vi "Smoothen Noise below Threshold.vi"(8 "Error In":errorcluster, 9 "Smoothing Width":dbl=1.0, 10 "Noise Threshold":dbl, 11 "Function in":dbl[](array[numeric])) -> (0 "Error Out":errorcluster, 3 "Function out":dbl[](array[numeric]))   [LabVIEW 2021, in "Arrays.lvlib"]
uses:
  Arrays.lvlib
  Linear Ramp End Options.ctl
  e7203b3f-f00a-46c5-81ee-9b5c31ab6268.vi
panel:
  out "Support Size":i32
  out "Waveform Graph":dbl[](graph)
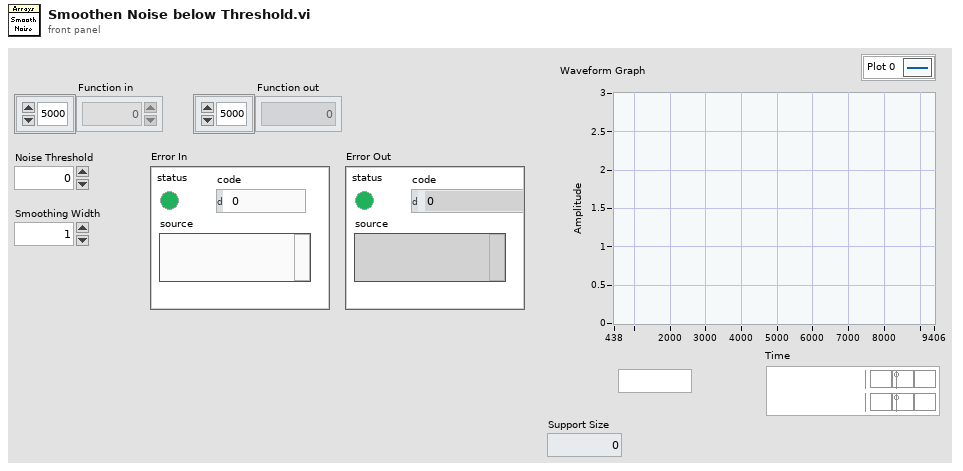
[diagram p1: front panel]
types:
  T1 = typedef "Arrays.lvlib/Linear Ramp End Options.ctl" = enum16{"Include Min/Exclude Max", "Exclude Min/Include Max", "Include Both Ends", "Exclude Both Ends"}
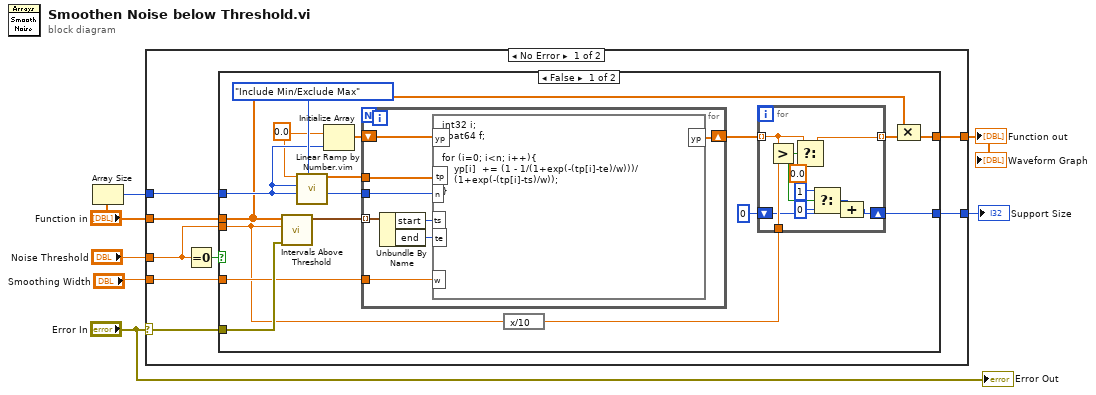
[diagram p0: block diagram]
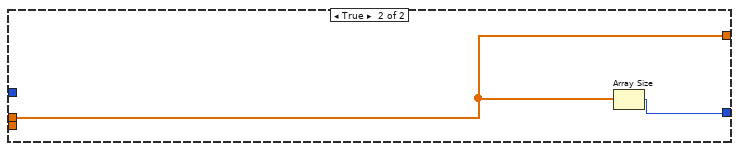
[diagram p2: hidden frame]
diagram:
  n1 = Array Size(array="Function in") -> (size(s)=w6:i32)
  n2 = case shown="No Error" "Error In" {
    selector: "Error In" -> [w15 _]
    tunnel: "Noise Threshold" -> [w11 _]
    tunnel: w6 -> [w12 _]
    tunnel: "Smoothing Width" -> [w14 _]
    tunnel: "Function in" -> [w8 w53]
    tunnel: [w13 w53] -> w2
    tunnel: [w9 _] -> w1
    frame No Error {
      n3 = Equal To 0?(x=w11) -> (x = 0?=w10:bool)
      n4 = case shown="False" w10 {
        tunnel: w15 -> [w32 _]
        tunnel: w14 -> [w30 _]
        tunnel: [w17 w52] -> w13
        tunnel: w8 -> [w16 w52]
        tunnel: w12 -> [w25 _]
        tunnel: w11 -> [w23 _]
        tunnel: [w18 w51] -> w9
        frame False {
          w24 = 0.0 ("size(s)")
          n5 = call "Intervals Above Threshold.vi"("Error In"=w32, "Noise Threshold"=w23, "Array in"=w16) -> ("Intervals above Threshold"=w27:cluster{"start":i32, "end":i32}[])  [unwired: 7 in, 1 out]
          n6 = call "Linear Ramp by Number.vim"("Options"=Linear_Ramp_End_Options."Include Min/Exclude Max", "# Steps (1)"=w25, "End (1)"=w25, "Start (0)"=w24) -> ("# Elements"=w28:i32, "Ramp"=w31:dbl[])  [unwired: 5 in, 1 out]
          n7 = Initialize Array(w24, w25) -> (w26:dbl[])
          n8 = for {
            tunnel: w27 -> [w48] mode=indexing
            tunnel: w31 -> [w50]
            tunnel: w28 -> [w49]
            tunnel: w30 -> [w45]
            shift-right: [w44] -> w22
            shift-left: w26 -> [w43]
            n9 = Unbundle By Name(w48) -> ("start"=w47:i32, "end"=w46:i32)
            n10 = formula code="int32 i;\nfloat64 f;\n\nfor (i=0; i<n; i++){\n    yp[i]  += (1 - 1/(1+exp(-(tp[i]-te)/w)))/\n    (1+exp(-(tp[i]-ts)/w));\n}"("tp"=w50, "n"=w49, "ts"=w47, "te"=w46, "w"=w45, "yp"=w43) -> ("yp"=w44:dbl[])
          }
          n11 = expression code="x/10"(w23) -> (w21:dbl)
          n12 = for {
            tunnel: w22 -> [w41] mode=indexing
            tunnel: w21 -> [w42]
            tunnel: [w39] -> w20 mode=indexing
            shift-right: [w37] -> w18
            shift-left: 0 -> [w38]
            n13 = Greater?(x=w41, y=w42) -> (0:w34:bool)
            n14 = Select(t=w41, s=w34, f=0.0) -> (s? t:f=w39:dbl)
            n15 = Select(t=1, s=w34, f=0) -> (s? t:f=w35:i32)
            n16 = Compound Arithmetic op=ADD(w35, w38) -> (w37:i32)
          }
          n17 = Compound Arithmetic op=MULTIPLY(w16, w20) -> (w17:dbl[])
        }
        frame True {
          n18 = Array Size(array=w52) -> (size(s)=w51:i32)
        }
      }
    }
    frame Error {
    }
  }
  "Function out" <- w2
  "Waveform Graph" <- w2
  "Support Size" <- w1
  "Error Out" <- "Error In"
